vi "UTILITY Read GEA Setup Data.vi"(8 "error in (no error)":errorcluster, 11 "General Startup Config Path":path) -> (0 "error out":errorcluster, 2 "Board Index":i32, 3 "Board ID":string)   [LabVIEW 2023]
uses:
  <vilib>/Utility/file.llb/Read Delimited Spreadsheet (string).vi
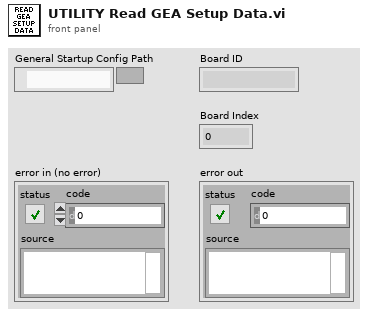
[diagram p1: front panel]
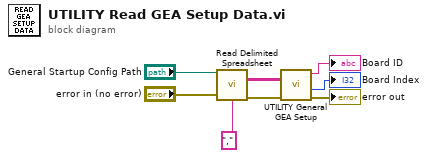
[diagram p0: block diagram]
diagram:
  n1 = call-poly <vilib>:"Read Delimited Spreadsheet.vi"("file path (dialog if empty)"="General Startup Config Path", "error in (no error)"="error in (no error)", "delimiter (\\t)"="," ("delimiter (\\t)")) -> ("all rows"=w6:string[][], "error out"=w2:errorcluster)  [unwired: 7 in, 4 out]
  n2 = call "UTILITY General GEA Setup.vi"("Error In"=w2, "all rows In"=w6) -> ("Error Out"=→"error out":errorcluster, "Board Index"=→"Board Index":i32, "Board ID"=→"Board ID":string)  [unwired: 6 in, 1 out]
